vi "Set Control Enabled State.vi"(7 "enabled (T)":bool=TRUE, 10 "error in (no error)":errorcluster, 11 "reference in":refnum<vi>) -> (2 "error out":errorcluster, 3 "reference out":refnum<vi>)   [LabVIEW 2020, in "varilib.lvlib"]
doc: "Change enabled state of the referenced control to 'Enabled' or 'Disabled and Grayed Out'. The status of the error in input is not important."
uses:
  varilib.lvlib
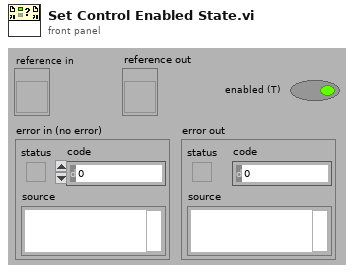
[diagram p1: front panel]
types:
  T1 = enum8{"Enabled", "Disabled", "Disabled and Grayed Out"}
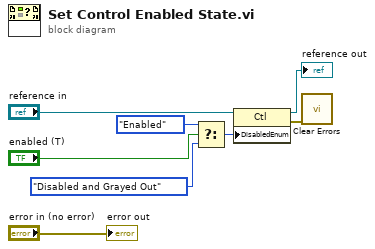
[diagram p0: block diagram]
diagram:
  n1 = Select(t=T1."Enabled" ("Disabled"), s="enabled (T)", f=T1."Disabled and Grayed Out" ("Disabled")) -> (s? t:f=w7:T1)
  n2 = property class="Ctl"(reference="reference in", "DisabledEnum"=w7) -> (reference out=→"reference out":refnum<vi>, error out=w3:errorcluster)  [unwired: 1 in]
  n3 = call <vilib>:"Clear Errors.vi"("error in (no error)"=w3) -> ()  [unwired: 5 in, 2 out]
  "error out" <- "error in (no error)"
